vi "Get Warning Position.vi"(7 "Warning":string) -> (3 "Warning position":i32)   [LabVIEW 2021, in "Converter.lvlib"]
uses:
  Converter.lvlib
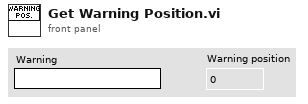
[diagram p1: front panel]
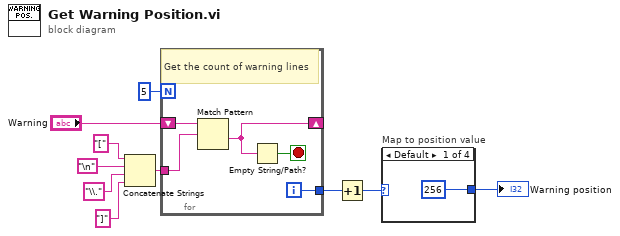
[diagram p0: block diagram]
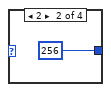
[diagram p2: hidden frame]
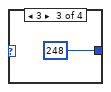
[diagram p3: hidden frame]
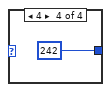
[diagram p4: hidden frame]
diagram:
  n1 = Concatenate Strings("[" ("string"), "\n", "\\." ("string"), "]" ("string")) -> (w9:string)
  n2 = for {
    N: 5 -> [_]
    tunnel: [w13] -> w10
    shift-right: [w12] -> _
    shift-left: "Warning" -> [w15]
    tunnel: w9 -> [w11]
    i -> [w13]
    stop <- w14 stop-if-true
    # "Get the count of warning lines"
    n3 = Match Pattern(string=w15, regular expression=w11) -> (after substring=w12:string)  [unwired: 1 in, 3 out]
    n4 = Empty String/Path?(string/path=w12) -> (empty?=w14:bool)
  }
  n5 = Increment(x=w10) -> (x+1=w2:i32)
  n6 = case "Map to position value" shown="Default" w2 {
    tunnel: [256 ("Warning position") 256 ("Warning position") 248 ("Warning position") 242 ("Warning position")] -> w1
    frame Default {
    }
    frame 2 {
    }
    frame 3 {
    }
    frame 4 {
    }
  }
  "Warning position" <- w1
